vi "Initialize.vi"(8 "error in":errorcluster, 10 "parameters":variant, 11 "SwitchDMM Channel in":refnum<class "SwitchDMM Channel.lvclass">) -> (0 "error out":errorcluster, 2 "summary":T1(array[cluster]), 3 "data value reference":refnum<data-value>)   [LabVIEW 2025, in "SwitchDMM Channel.lvclass"]
doc: "Initializes the data of a node to its default state.\nThe object is not created inside of this VI, because it is created from a File depending on user selection.\nCopyright 2017 National Instruments Corporation\n\nLicensed under the Apache License, Version 2.0 (the \"License\"); you may not use this file except in compliance with the License. You may obtain a copy of the License at http://www.apache.org/licenses/LICENSE-2.0\nUnless required by applicable law or agreed to in writing, software distributed under the License is distributed on an \"AS IS\" BASIS, WITHOUT WARRANTIES OR CONDITIONS OF ANY KIND, either express or implied. See the License for the specific language governing permissions and limitations under the License."
uses:
  SwitchDMM Channel.lvclass
  C:/Users/Public/Documents/Sandia National Labs/TSS Plugin/CEF.lvlibp/Node/CEF_Node.lvclass
  Users/Public/Documents/Sandia National Labs/TSS Plugin/CEF.lvlibp/Node/CEF_Node.lvclass
  DMM Instrument/DMM Instrument.lvclass
  SwitchDMM Channel.lvclass/SwitchDMM Channel.ctl
  DMM configuration/DMM configuration.lvclass
  C:/Users/Public/Documents/Sandia National Labs/TSS Plugin/Abstract Engine.lvlibp/Plugin/Abstract/Instrument configuration/Instrument configuration.lvclass
  SwitchDMM Channel configuration/SwitchDMM Channel configuration.lvclass
  C:/Users/Public/Documents/Sandia National Labs/TSS Plugin/Abstract Engine.lvlibp/Plugin/Abstract/Channel configuration/Channel configuration.lvclass
  Users/Public/Documents/Sandia National Labs/TSS Plugin/CEF.lvlibp/Node/ReadParent.vi
  Users/Public/Documents/Sandia National Labs/TSS Plugin/CEF.lvlibp/Node/ReadChildren.vi
  Users/Public/Documents/Sandia National Labs/TSS Plugin/Abstract Engine.lvlibp/Plugin/Abstract/Instrument configuration/Read Instrument Setting.vi
  Users/Public/Documents/Sandia National Labs/TSS Plugin/Abstract Engine.lvlibp/Plugin/Abstract/Channel configuration/Read Channel Setting.vi
  Users/Public/Documents/Sandia National Labs/TSS Plugin/Abstract Engine.lvlibp/Plugin/Abstract/Channel configuration/Write Channel Setting.vi
  Users/Public/Documents/Sandia National Labs/TSS Plugin/CEF.lvlibp/serializable configuration/CEF_serializable configuration.lvclass
  Users/Public/Documents/Sandia National Labs/TSS Plugin/Abstract Engine.lvlibp/Plugin/Abstract/Abstract Channel/Abstract Channel.lvclass
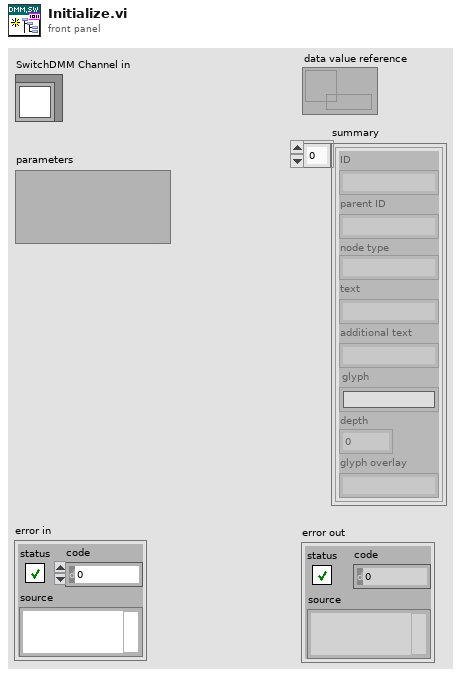
[diagram p1: front panel]
types:
  T1 = cluster{"ID":string, "parent ID":string, "node type":string, "text":string, "additional text":string, "glyph":string, "depth":i32, "glyph overlay":string}[]
  T2 = typedef "Abstract Engine.lvlibp/Instrument configuration.lvclass/Default Instrument.ctl" = cluster{"Type":string, "Address":string, "SW Alias":string, "Description":string, "Enabled":bool}
  T3 = typedef "Abstract Engine.lvlibp/Channel configuration.lvclass/Default Channel.ctl" = cluster{"Address":string, "SW Alias":string, "Enabled":bool, "Type":string, "Description":string}
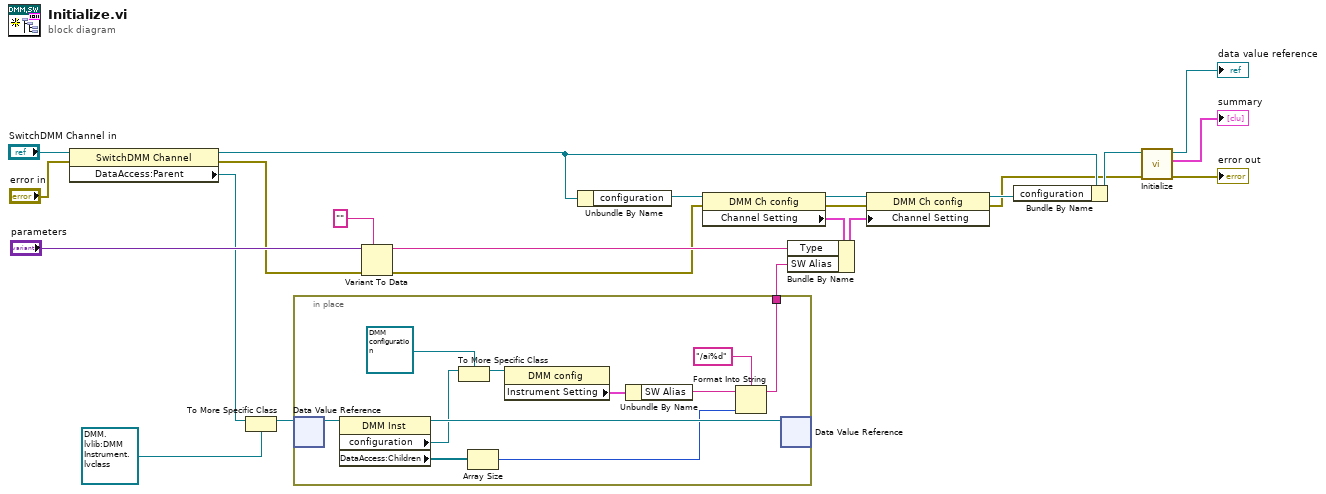
[diagram p0: block diagram]
diagram:
  n1 = property class="SwitchDMM Channel"(reference="SwitchDMM Channel in", error in="error in") -> (reference out=w18:refnum<class "SwitchDMM Channel.lvclass">, error out=w12:errorcluster, "DataAccess:Parent"=w9:refnum<data-value>)
  n2 = To More Specific Class(target class=refnum<data-value> refnum ("data value reference"), reference=w9) -> (specific class reference=w8:refnum<data-value>)  [unwired: 1 in, 1 out]
  n3 = in-place {
    in-place-border: [w32] -> w7
    n4 = in-place-dvr #1(w8) -> (w31:refnum<class "DMM Instrument.lvclass">)  [unwired: 1 out]
    n5 = property class="DMM Inst"(reference=w31) -> (reference out=w30:refnum<class "DMM Instrument.lvclass">, "configuration"=w29:refnum<class "CEF_serializable configuration.lvclass">, "DataAccess:Children"=w28:refnum<data-value>[])  [unwired: 1 in, 1 out]
    n6 = To More Specific Class(target class=refnum<class "DMM configuration.lvclass"> refnum ("DMM.lvlib:DMM config"), reference=w29) -> (specific class reference=w26:refnum<class "DMM configuration.lvclass">)  [unwired: 1 in, 1 out]
    n7 = Array Size(array=w28) -> (size(s)=w27:i32)
    n8 = property class="DMM config"(reference=w26) -> ("Instrument Setting"=w25:T2)  [unwired: 1 in, 2 out]
    n9 = Unbundle By Name(w25) -> ("SW Alias"=w34:string)
    n10 = Format Into String(format string="/ai%d", initial string=w34, w27) -> (resulting string=w32:string)  [unwired: 1 in, 1 out]
    n11 = in-place-dvr #1(w30) -> ()  [unwired: 2 out]
  }
  n12 = Variant To Data(error in=w12, type="", Variant="parameters") -> (data=w15:string, error out=w11:errorcluster)
  n13 = Unbundle By Name(w18) -> ("configuration"=w19:refnum<class "SwitchDMM Channel configuration.lvclass">)
  n14 = property class="DMM Ch config"(reference=w19, error in=w11) -> (reference out=w5:refnum<class "SwitchDMM Channel configuration.lvclass">, error out=w10:errorcluster, "Channel Setting"=w3:T3)
  n15 = Bundle By Name(cluster=w3, "Type"=w15, "SW Alias"=w7) -> (w4:T3)
  n16 = property class="DMM Ch config"(reference=w5, error in=w10, "Channel Setting"=w4) -> (reference out=w16:refnum<class "SwitchDMM Channel configuration.lvclass">, error out=w6:errorcluster)
  n17 = Bundle By Name(cluster=w18, "configuration"=w16) -> (w17:refnum<class "SwitchDMM Channel.lvclass">)
  n18 = call-parent "Initialize.vi"("error in"=w6, "CEF_Serialize node in"=w17) -> ("error out"=→"error out":errorcluster, "summary"=→"summary":T1, "data value reference"=→"data value reference":refnum<data-value>)  [unwired: 7 in]
